vi "Write Child XML Node.vi"(8 "error in (no error)":errorcluster, 10 "Child XML Node":refnum<k20>, 11 "Array in":refnum<class "Array.lvclass">) -> (0 "error out":errorcluster, 3 "Array out":refnum<class "Array.lvclass">)   [LabVIEW 2025, in "Array.lvclass"]
uses:
  Array.lvclass
  Array.lvclass/Array.ctl
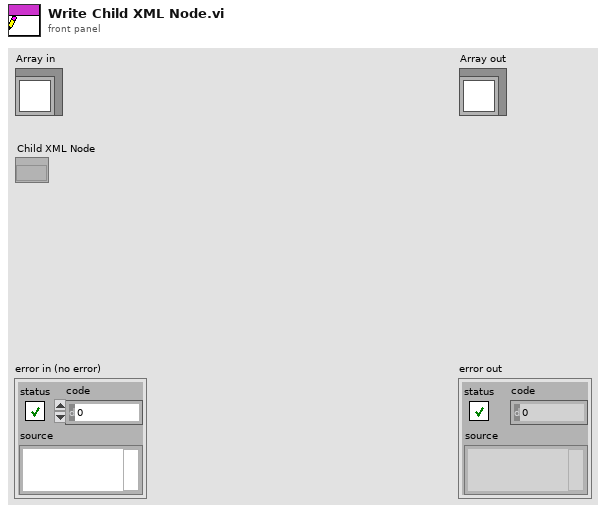
[diagram p1: front panel]
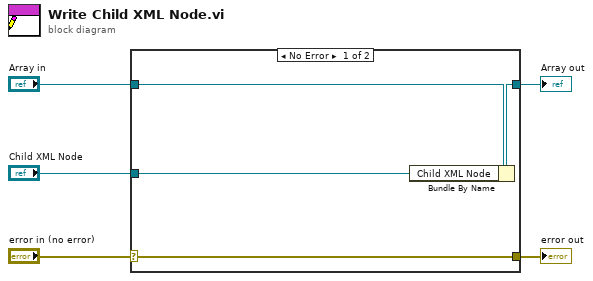
[diagram p0: block diagram]
diagram:
  n1 = case shown="No Error" "error in (no error)" {
    selector: "error in (no error)" -> [w9 w10]
    tunnel: [w9 w10] -> w4
    tunnel: [w7 w11] -> w2
    tunnel: "Array in" -> [w8 w11]
    tunnel: "Child XML Node" -> [w6 _]
    frame No Error {
      n2 = Bundle By Name(cluster=w8, "Child XML Node"=w6) -> (w7:refnum<class "Array.lvclass">)
    }
    frame Error {
    }
  }
  "error out" <- w4
  "Array out" <- w2
